vi "OMEGA_Load_Analog.vi"(6 "channel":T1) -> ()   [LabVIEW 2020]
doc: "I. Description:\nThis example demonstrates how to continuously acquire data (Waveform) using the DAQ device's internal clock and an analog slope start trigger.\n\nII. Instructions for Running:\n1. Select the physical channel to correspond to where your signal is input on the DAQ device.\n2. Enter the minimum and maximum voltage ranges.\nNote: For better accuracy try to match the Input Ranges to the expected voltage level of the measured signal.\n3. Set the rate of the acquisition. Also set the Samples to Read control. This will determine how many samples are read each time the while loop iterates. This also determines how many points are plotted on the graph each iteration.\nNote: The rate should be at least twice as fast as the maximum frequency component of the signal being acquired.\n4. Set the source of the Analog Slope Start Trigger.\n5. Set the slope and level of desired analog edge condition.\n\nIII. Block Diagram Steps:\n1. Create an analog input voltage channel.\n2. Set the rate for the sample clock. Additionally, define the sample mode to be continuous.\n3. Define the parameters for an Analog Slope Start Trigger.\n4. Call the Start VI to start the acquisition.\n5. Read the waveform data in a loop until the user hits the stop button or an error occurs.\n6. Call the Clear Task VI to clear the Task.\n7. Use the popup dialog box to display an error if any.\n\nIV. I/O Connections Overview:\nMake sure your signal input terminal matches the Physical Channel I/O control. Also, make sure your analog trigger terminal matches the Trigger Source Control. For further connection information, refer to your hardware reference manual."
uses:
  <extravilib>/ChannelInstances/Tag-bool/))Channel.ctl
  <vilib>/Utility/error.llb/DialogType.ctl
  <extravilib>/ChannelInstances/Tag-bool/Read With Abort.vi
  <vilib>/ULx/Create Channel.llb/ULx Create Channel (AI-Voltage-Basic).vi
  <vilib>/ULx/Timing.llb/ULx Timing (Sample Clock).vi
  <extravilib>/ChannelInstances/Tag-bool/EndpointRead.vi
  <vilib>/ULx/Read.llb/ULx Read (Analog 1D Wfm NChan NSamp).vi
  <extravilib>/ChannelInstances/Tag-bool.lvlib
panel:
  out "Waveform Graph":waveform(dbl)[](graph)
  in  "maximum value":dbl=5.0
  in  "minimum value":dbl=-5.0
  # "For instructions, select Help>>Show Context Help"
  # "Channel Parameters"
  # "* Please refer to your device documentation for information \nregarding valid Analog Triggers for your device."
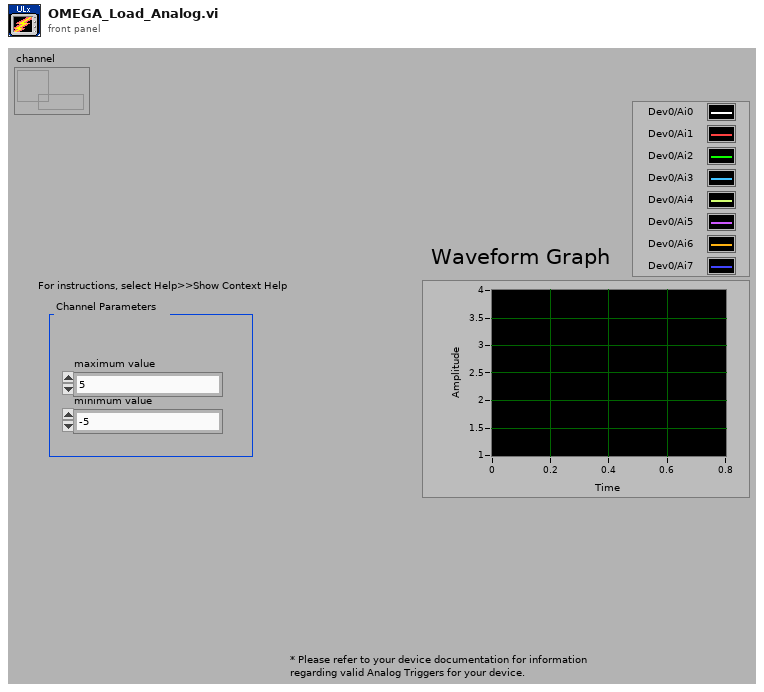
[diagram p1: front panel]
types:
  T1 = typedef "Tag-bool.lvlib/))Channel.ctl" = refnum<queue>
  T2 = typedef "DialogType.ctl" = u16
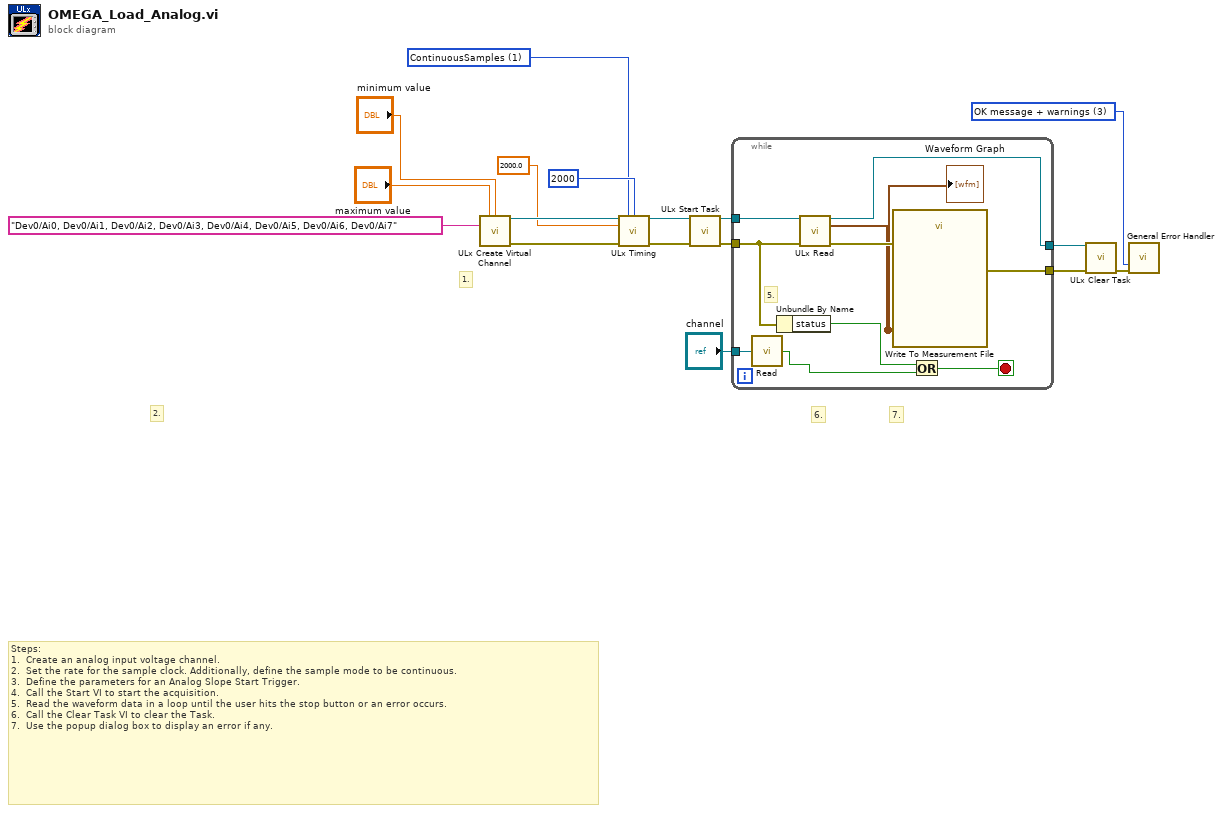
[diagram p0: block diagram]
diagram:
  w3 = 1 items=["FiniteSamples", "ContinuousSamples"] ("sample mode")
  w10 = T2 3 items=["no dialog", "OK message", "continue or stop message", "OK message + warnings", "continue/stop + warnings"] ("type of dialog (OK msg:1)")
  # "7."
  # "6."
  # "Steps: \n1.  Create an analog input voltage channel.\n2.  Set the rate for the sample clock. Additionally, define the sample mode to be continuous.\n3.  Define the parameters for an Analog Slope Start Trigger.\n4.  Call the Start VI to start the acquisition.\n5.  Read the waveform data in a loop until the user hits the stop button or an error occurs.\n6.  Call the Clear Task VI to clear the Task.\n7.  Use the popup dialog box to display an error if any."
  # "2."
  # "1."
  n1 = call-poly <vilib>:"ULx Create Virtual Channel.vi"("maximum value"="maximum value", "minimum value"="minimum value", "physical channels"="Dev0/Ai0, Dev0/Ai1, Dev0/Ai2, Dev0/Ai3, Dev0/Ai4, Dev0/Ai5, Dev0/Ai6, Dev0/Ai7") -> ("task out"=w14:refnum<k24>, "error out"=w17:errorcluster)  [unwired: 11 in]
  n2 = call-poly <vilib>:"ULx Timing.vi"("task in"=w14, "sample mode"=w3, "samples per channel"=2000, "rate"=2000.0, "error in"=w17) -> ("task out"=w9:refnum<k24>, "error out"=w8:errorcluster)  [unwired: 9 in]
  n3 = call <vilib>:"ULx Start Task.vi"("task in"=w9, "error in"=w8) -> ("task out"=w13:refnum<k24>, "error out"=w16:errorcluster)  [unwired: 12 in]
  n4 = while {
    tunnel: w16 -> [w21]
    tunnel: w13 -> [w27]
    tunnel: [w26] -> w12
    tunnel: [w22] -> w11
    tunnel: "channel" -> [w18]
    stop <- w24 stop-if-true
    # "5."
    n5 = call <extravilib>:"Read.vi"("channel"=w18) -> ("element"=w19:bool)  [unwired: 1 in, 1 out]
    n6 = Unbundle By Name(w21) -> ("status"=w25:bool)
    n7 = call-poly <vilib>:"ULx Read.vi"("task in"=w27, "error in"=w21) -> ("task out"=w26:refnum<k24>, "data"=w20:waveform(dbl)[], "error out"=w23:errorcluster)  [unwired: 11 in]
    "Waveform Graph" <- w20
    n8 = call "Write To Measurement File"("Signals"=w20, "error in (no error)"=w23) -> ("error out"=w22:errorcluster)  [unwired: 15 in, 2 out]
    n9 = Or(x=w25, y=w19) -> (x .or. y?=w24:bool)
  }
  n10 = call <vilib>:"ULx Clear Task.vi"("task in"=w12, "error in"=w11) -> ("error out"=w15:errorcluster)  [unwired: 13 in]
  n11 = call <vilib>:"General Error Handler.vi"("type of dialog (OK msg:1)"=w10, "error in (no error)"=w15) -> ()  [unwired: 9 in, 5 out]
